vi "Agilent ENA Series Interactive Application.vi"() -> ()   [LabVIEW 2011]
doc: "This VI illustrates typical measuring task for a network analyzer. The described measured task is transmission measurement of magnitude and phase."
panel:
  in  "Save State (F: Disable)":bool
  in  "Power (dBm)":dbl=-10.0 format="%^.2e"
  in  "IF Bandwidth":dbl=10000.0 format="%^.2e"
  in  "Span Frequency [Hz]":dbl=200000000.0 format="%^.2e"
  in  "Center Frequency [Hz]":dbl=947500000.0 format="%^.2e"
  in  "VISA resource name":refnum<visa-resource-name>
  # "(c) 2005-2015 National Instruments.  ALL RIGHTS RESERVED."
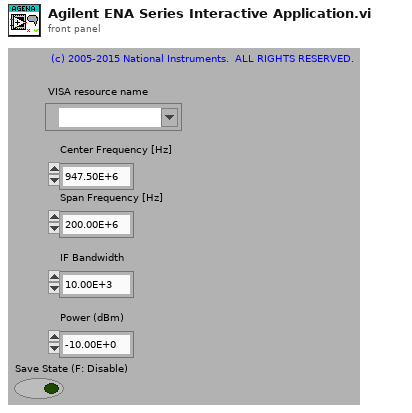
[diagram p1: front panel]
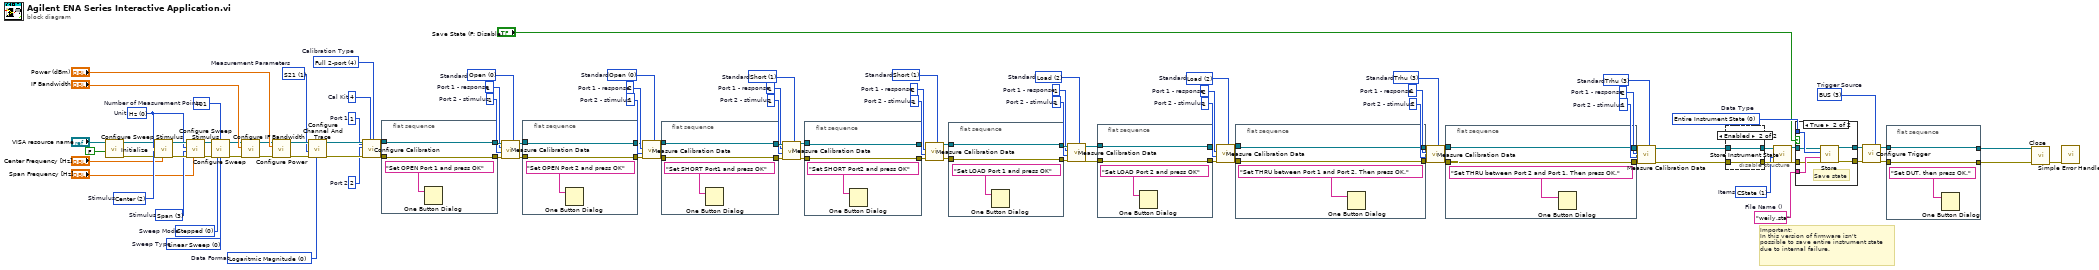
[diagram p0: block diagram]
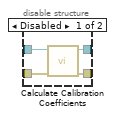
[diagram p2: hidden frame]
diagram:
  w24 = u16 3 items=["Internal", "External", "Manual", "BUS"]  # Trigger Source
  w16 = "weily.sta"  # File Name ()
  w17 = u16 0 items=["Entire Instrument State", "Formatted Data Array", "Image On The LCD Display", "Segment Sweep Table", "Limit Table", "Power Sensor A", "Power Sensor B", "VBA Project", "Loss Compensation Table 1", "Loss Compensation Table 2", "Loss Compensation Table 3", "Loss Compensation Table 4"]  # Data Type
  w3 = u16 1 items=["State", "CState", "Dstate", "CDState"]  # Items
  w27 = u16 3 items=["Open", "Short", "Load", "Trhu", "Isolation"]  # Standard
  w29 = 1  # Port 2 - stimulus
  w28 = 2  # Port 1 - response
  w36 = u16 3 items=["Open", "Short", "Load", "Trhu", "Isolation"]  # Standard
  w32 = 2  # Port 2 - stimulus
  w33 = 1  # Port 1 - response
  w39 = u16 2 items=["Open", "Short", "Load", "Trhu", "Isolation"]  # Standard
  w43 = 1  # Port 2 - stimulus
  w42 = 2  # Port 1 - response
  w50 = u16 2 items=["Open", "Short", "Load", "Trhu", "Isolation"]  # Standard
  w46 = 1  # Port 2 - stimulus
  w47 = 1  # Port 1 - response
  w53 = u16 1 items=["Open", "Short", "Load", "Trhu", "Isolation"]  # Standard
  w57 = 1  # Port 2 - stimulus
  w56 = 2  # Port 1 - response
  w64 = u16 1 items=["Open", "Short", "Load", "Trhu", "Isolation"]  # Standard
  w60 = 1  # Port 2 - stimulus
  w61 = 1  # Port 1 - response
  w65 = u16 0 items=["Open", "Short", "Load", "Trhu", "Isolation"]  # Standard
  w66 = u16 0 items=["Open", "Short", "Load", "Trhu", "Isolation"]  # Standard
  w72 = 1  # Port 2 - stimulus
  w71 = 2  # Port 1 - response
  w73 = 1  # Port 2 - stimulus
  w74 = 1  # Port 1 - response
  w79 = 2  # Port 2
  w80 = 1  # Port 1
  w81 = u16 4 items=["Open", "Short", "Through", "1-port", "Full 2-port", "Full 3-port", "Full 4-port"]  # Calibration Type
  w82 = 4  # Cal Kit
  w85 = u16 0 items=["Logaritmic Magnitude", "Phase", "Group Delay", "Smith Chart  Linear (Lin/Phase)", "Smith Chart  Logaritmic (Log/Phase)", "Smith Chart  Complex (Real/Imag)", "Smith Chart  Impedance (R+jX)", "Smith Chart  Admittance (G+jB)", "Polar Format (Linear)", "Polar Format (Logaritmic)", "Polar Format (Re/Im)", "Linear Magnitude", "SWR", "Real", "Imaginary", "Epanded Phase", "Positive Phase"]  # Data Format
  w86 = u16 1 items=["S11", "S21", "S31", "S41", "S12", "S22", "S32", "S42", "S13", "S23", "S33", "S43", "S14", "S24", "S34", "S44", "A", "B", "C", "D", "R1", "R2", "R3", "R4"]  # Measurement Parameters
  w97 = u16 0 items=["Linear Sweep", "Logaritmic Sweep", "Segment Sweep", "Power Sweep"]  # Sweep Type
  w98 = 401  # Number of Measurement Points
  w99 = u16 0 items=["Stepped", "Swept", "Fast Stepped Mode", "Fast Swept Mode"]  # Sweep Mode
  w102 = u16 3 items=["Start", "Stop", "Center", "Span"]  # Stimulus
  w100 = u16 0 items=["Hz", "kHz", "MHz", "GHz", "dBm", "s"]  # Unit
  w106 = u16 2 items=["Start", "Stop", "Center", "Span"]  # Stimulus
  # "Important:\nIn this version of firmware isn't \npossible to save entire instrument state\ndue to internal failure."
  n1 = call "Initialize.vi"("Reset? (T: Yes)"=FALSE, "VISA resource name"="VISA resource name") -> ("error out"=w18:errorcluster, "VISA resource name out"=w19:refnum<visa-resource-name>)  [unwired: 8 in]
  n2 = call "Configure Sweep Stimulus.vi"("Parameter (0.0)"="Center Frequency [Hz]", "error in (no error)"=w18, "Stimulus (0: Start)"=w106, "Unit (0: Hz)"=w100, "VISA resource name"=w19) -> ("error out"=w104:errorcluster, "VISA resource name out"=w103:refnum<visa-resource-name>)  [unwired: 5 in]
  n3 = call "Configure Sweep Stimulus.vi"("Parameter (0.0)"="Span Frequency [Hz]", "error in (no error)"=w104, "Stimulus (0: Start)"=w102, "Unit (0: Hz)"=w100, "VISA resource name"=w103) -> ("error out"=w96:errorcluster, "VISA resource name out"=w95:refnum<visa-resource-name>)  [unwired: 5 in]
  n4 = call "Configure Sweep.vi"("VISA resource name"=w95, "Number of Measurement Points (201)"=w98, "error in (no error)"=w96, "Sweep Mode (0: Stepped)"=w99, "Sweep Type (0: Linear Sweep)"=w97) -> ("VISA resource name out"=w93:refnum<visa-resource-name>, "error out"=w92:errorcluster)  [unwired: 9 in]
  n5 = call "Configure IF Bandwidth.vi"("error in (no error)"=w92, "IF Bandwidth (100000.0)"="IF Bandwidth", "VISA resource name"=w93) -> ("error out"=w90:errorcluster, "VISA resource name out"=w89:refnum<visa-resource-name>)  [unwired: 7 in]
  n6 = call "Configure Power.vi"("VISA resource name"=w89, "Power Level (0.0)"="Power (dBm)", "error in (no error)"=w90) -> ("VISA resource name out"=w88:refnum<visa-resource-name>, "error out"=w87:errorcluster)  [unwired: 11 in]
  n7 = call "Configure Channel And Trace.vi"("Data Format (0: Logarithmic Magnitude)"=w85, "error in (no error)"=w87, "Measurement Parameters (0: S11)"=w86, "VISA resource name"=w88) -> ("error out"=w83:errorcluster, "VISA resource name out"=w84:refnum<visa-resource-name>)  [unwired: 6 in]
  n8 = call "Configure Calibration.vi"("VISA resource name"=w84, "Port 1 (1)"=w80, "Port 2 (1)"=w79, "error in (no error)"=w83, "Cal Kit (1)"=w82, "Calibration Type (6: Full 4-port)"=w81) -> ("VISA resource name out"=w78:refnum<visa-resource-name>, "error out"=w77:errorcluster)  [unwired: 12 in]
  n9 = flat-sequence {
    tunnel: w78 -> [w108]
    tunnel: w77 -> [w107]
    tunnel: [w107] -> w75
    tunnel: [w108] -> w76
    frame #0 {
      n10 = One Button Dialog(message="Set OPEN Port 1 and press OK") -> ()  [unwired: 1 in, 1 out]
    }
  }
  n11 = call "Measure Calibration Data.vi"("Standard (0: Open)"=w66, "error in (no error)"=w75, "Port 2 - stimulus (2)"=w73, "Port 1 - response (1)"=w74, "VISA resource name"=w76) -> ("error out"=w67:errorcluster, "VISA resource name out"=w68:refnum<visa-resource-name>)  [unwired: 5 in]
  n12 = flat-sequence {
    tunnel: w68 -> [w111]
    tunnel: w67 -> [w110]
    tunnel: [w110] -> w70
    tunnel: [w111] -> w69
    frame #0 {
      n13 = One Button Dialog(message="Set OPEN Port 2 and press OK") -> ()  [unwired: 1 in, 1 out]
    }
  }
  n14 = call "Measure Calibration Data.vi"("Standard (0: Open)"=w65, "error in (no error)"=w70, "Port 2 - stimulus (2)"=w72, "Port 1 - response (1)"=w71, "VISA resource name"=w69) -> ("error out"=w58:errorcluster, "VISA resource name out"=w59:refnum<visa-resource-name>)  [unwired: 5 in]
  n15 = flat-sequence {
    tunnel: w59 -> [w114]
    tunnel: w58 -> [w113]
    tunnel: [w113] -> w62
    tunnel: [w114] -> w63
    frame #0 {
      n16 = One Button Dialog(message="Set SHORT Port1 and press OK") -> ()  [unwired: 1 in, 1 out]
    }
  }
  n17 = call "Measure Calibration Data.vi"("Standard (0: Open)"=w64, "error in (no error)"=w62, "Port 2 - stimulus (2)"=w60, "Port 1 - response (1)"=w61, "VISA resource name"=w63) -> ("error out"=w51:errorcluster, "VISA resource name out"=w52:refnum<visa-resource-name>)  [unwired: 5 in]
  n18 = flat-sequence {
    tunnel: w52 -> [w117]
    tunnel: w51 -> [w116]
    tunnel: [w116] -> w55
    tunnel: [w117] -> w54
    frame #0 {
      n19 = One Button Dialog(message="Set SHORT Port2 and press OK") -> ()  [unwired: 1 in, 1 out]
    }
  }
  n20 = call "Measure Calibration Data.vi"("Standard (0: Open)"=w53, "error in (no error)"=w55, "Port 2 - stimulus (2)"=w57, "Port 1 - response (1)"=w56, "VISA resource name"=w54) -> ("error out"=w44:errorcluster, "VISA resource name out"=w45:refnum<visa-resource-name>)  [unwired: 5 in]
  n21 = flat-sequence {
    tunnel: w45 -> [w120]
    tunnel: w44 -> [w119]
    tunnel: [w119] -> w48
    tunnel: [w120] -> w49
    frame #0 {
      n22 = One Button Dialog(message="Set LOAD Port 1 and press OK") -> ()  [unwired: 1 in, 1 out]
    }
  }
  n23 = call "Measure Calibration Data.vi"("Standard (0: Open)"=w50, "error in (no error)"=w48, "Port 2 - stimulus (2)"=w46, "Port 1 - response (1)"=w47, "VISA resource name"=w49) -> ("error out"=w37:errorcluster, "VISA resource name out"=w38:refnum<visa-resource-name>)  [unwired: 5 in]
  n24 = flat-sequence {
    tunnel: w38 -> [w123]
    tunnel: w37 -> [w122]
    tunnel: [w122] -> w41
    tunnel: [w123] -> w40
    frame #0 {
      n25 = One Button Dialog(message="Set LOAD Port 2 and press OK") -> ()  [unwired: 1 in, 1 out]
    }
  }
  n26 = call "Measure Calibration Data.vi"("Standard (0: Open)"=w39, "error in (no error)"=w41, "Port 2 - stimulus (2)"=w43, "Port 1 - response (1)"=w42, "VISA resource name"=w40) -> ("error out"=w30:errorcluster, "VISA resource name out"=w31:refnum<visa-resource-name>)  [unwired: 5 in]
  n27 = flat-sequence {
    tunnel: w31 -> [w126]
    tunnel: w30 -> [w125]
    tunnel: [w125] -> w34
    tunnel: [w126] -> w35
    frame #0 {
      n28 = One Button Dialog(message="Set THRU between Port 1 and Port 2. Then press OK.") -> ()  [unwired: 1 in, 1 out]
    }
  }
  n29 = call "Measure Calibration Data.vi"("Standard (0: Open)"=w36, "error in (no error)"=w34, "Port 2 - stimulus (2)"=w32, "Port 1 - response (1)"=w33, "VISA resource name"=w35) -> ("error out"=w25:errorcluster, "VISA resource name out"=w26:refnum<visa-resource-name>)  [unwired: 5 in]
  n30 = flat-sequence {
    tunnel: w26 -> [w129]
    tunnel: w25 -> [w128]
    tunnel: [w128] -> w11
    tunnel: [w129] -> w12
    frame #0 {
      n31 = One Button Dialog(message="Set THRU between Port 2 and Port 1. Then press OK.") -> ()  [unwired: 1 in, 1 out]
    }
  }
  n32 = call "Measure Calibration Data.vi"("Standard (0: Open)"=w27, "error in (no error)"=w11, "Port 2 - stimulus (2)"=w29, "Port 1 - response (1)"=w28, "VISA resource name"=w12) -> ("error out"=w8:errorcluster, "VISA resource name out"=w9:refnum<visa-resource-name>)  [unwired: 5 in]
  n33 = disable-structure shown="Enabled" {
    disable-tunnel: w9 -> [w134 w136]
    disable-tunnel: w8 -> [w133 w135]
    disable-tunnel: [w132 w135] -> w7
    disable-tunnel: [w131 w136] -> w6
    frame Disabled {
      n34 = call "Calculate Calibration Coefficients.vi"("error in (no error)"=w133, "VISA resource name"=w134) -> ("error out"=w132:errorcluster, "VISA resource name out"=w131:refnum<visa-resource-name>)  [unwired: 8 in]
    }
    frame Enabled {
    }
  }
  n35 = call "Store Instrument State.vi"("error in (no error)"=w7, "Items (1: CState)"=w3, "VISA resource name"=w6) -> ("error out"=w4:errorcluster, "VISA resource name out"=w5:refnum<visa-resource-name>)  [unwired: 7 in]
  n36 = case shown="True" "Save State (F: Disable)" {
    tunnel: w17 -> [_ w144]
    tunnel: w16 -> [_ w143]
    tunnel: w5 -> [w138 w142]
    tunnel: [w138 w141] -> w15
    tunnel: w4 -> [w137 w140]
    tunnel: [w137 w139] -> w14
    frame False {
      # "Don't save"
    }
    frame True {
      # "Save state"
      n37 = call "Store.vi"("error in (no error)"=w140, "File Name ()"=w143, "Data Type (0: Entire Instrument State)"=w144, "VISA resource name"=w142) -> ("error out"=w139:errorcluster, "VISA resource name out"=w141:refnum<visa-resource-name>)  [unwired: 6 in]
    }
  }
  n38 = call "Configure Trigger.vi"("Trigger Source (0: Internal)"=w24, "error in (no error)"=w14, "VISA resource name"=w15) -> ("error out"=w22:errorcluster, "VISA resource name out"=w23:refnum<visa-resource-name>)  [unwired: 7 in]
  n39 = flat-sequence {
    tunnel: w23 -> [w145]
    tunnel: w22 -> [w146]
    tunnel: [w146] -> w1
    tunnel: [w145] -> w2
    frame #0 {
      n40 = One Button Dialog(message="Set DUT, then press OK.") -> ()  [unwired: 1 in, 1 out]
    }
  }
  n41 = call "Close.vi"("error in (no error)"=w1, "VISA resource name"=w2) -> ("error out"=w21:errorcluster)  [unwired: 9 in]
  n42 = call <vilib>:"Simple Error Handler.vi"("error in (no error)"=w21) -> ()  [unwired: 4 in, 5 out]
